vi "Delete Password.vi"(8 "error in (no error)":errorcluster, 10 "index":i32, 11 "Master in":refnum<class "MASTER.lvclass">) -> (0 "error out":errorcluster, 3 "Master out":refnum<class "MASTER.lvclass">)   [LabVIEW 2014, in "Files Library.lvlib" / "Master.lvclass"]
uses:
  MASTER/MASTER.lvclass
  MASTER/MASTER.lvclass/MASTER.ctl
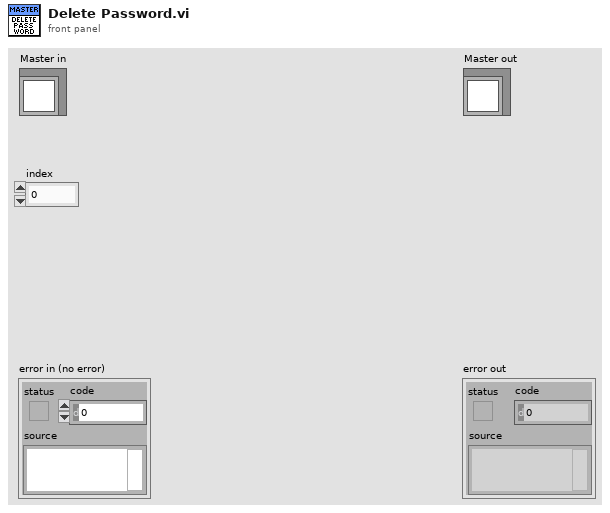
[diagram p1: front panel]
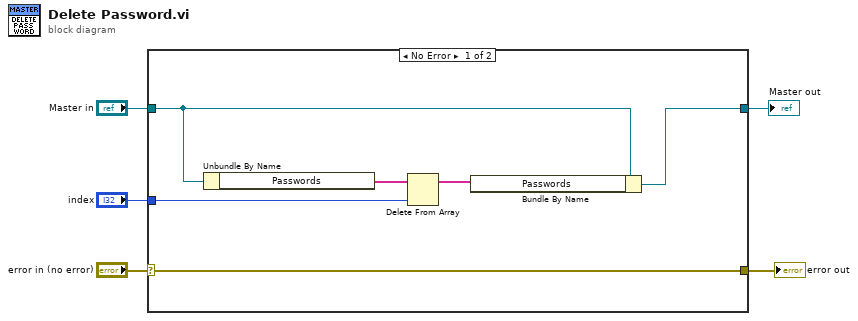
[diagram p0: block diagram]
diagram:
  n1 = case shown="No Error" "error in (no error)" {
    selector: "error in (no error)" -> [w11 w13]
    tunnel: [w11 w13] -> w4
    tunnel: [w8 w12] -> w2
    tunnel: "Master in" -> [w9 w12]
    tunnel: "index" -> [w6 _]
    frame No Error {
      n2 = Unbundle By Name(w9) -> ("Passwords"=w10:string[])
      n3 = Delete From Array(array=w10, index=w6) -> (array with subset deleted=w7:string[])  [unwired: 1 in, 1 out]
      n4 = Bundle By Name(cluster=w9, "Passwords"=w7) -> (w8:refnum<class "MASTER.lvclass">)
    }
    frame Error {
    }
  }
  "error out" <- w4
  "Master out" <- w2
